vi "SPIN2_ODFT_iHV_w_Programmable_Delay.vi"(7 "Delay Time (s)":dbl=0.001 format="%#_13p", 9 "script name":string="ODFTwHV0", 10 "Ext_HV":dbl=38.0 format="%#_13g", 11 "Semiconductor Module Context":T1) -> (0 "error out":errorcluster)   [LabVIEW 2013]
uses:
  <vilib>/NI_TestStand_SemiconductorModule/NI_TestStand_Semiconductor_Module.lvlibp/PinMap/General/SemiconductorModuleContext.ctl
  <instrlib>/niHSDIO/niHSDIO.llb/niHSDIO_ctl Trigger Script - trigID Values (Ring).ctl
  <vilib>/NI_TestStand_SemiconductorModule/NI_TestStand_Semiconductor_Module.lvlibp/PinMap/DC Power/PinsToNIDCPowerSessions.vi
  <vilib>/NI_TestStand_SemiconductorModule/NI_TestStand_Semiconductor_Module.lvlibp/PinMap/Deprecated/PublishDataDoubleMultiplePinsMultipleInstruments.vi
  <vilib>/NI_TestStand_SemiconductorModule/NI_TestStand_Semiconductor_Module.lvlibp
panel:
  out "current measurements":dbl[][](array[numeric])
  out "Delta_iHV_Measurements":dbl[][](array[numeric])
  in  "Pins":string[](array[string])=["HV"]
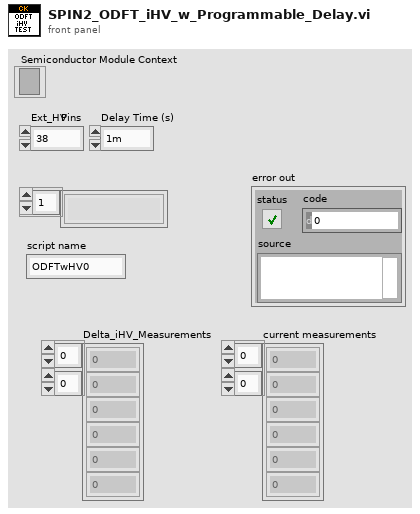
[diagram p1: front panel]
types:
  T1 = typedef "NI_TestStand_Semiconductor_Module.lvlibp/SemiconductorModuleContext.ctl" = refnum<k7>
  T2 = typedef "niHSDIO_ctl Trigger Script - trigID Values (Ring).ctl" = string
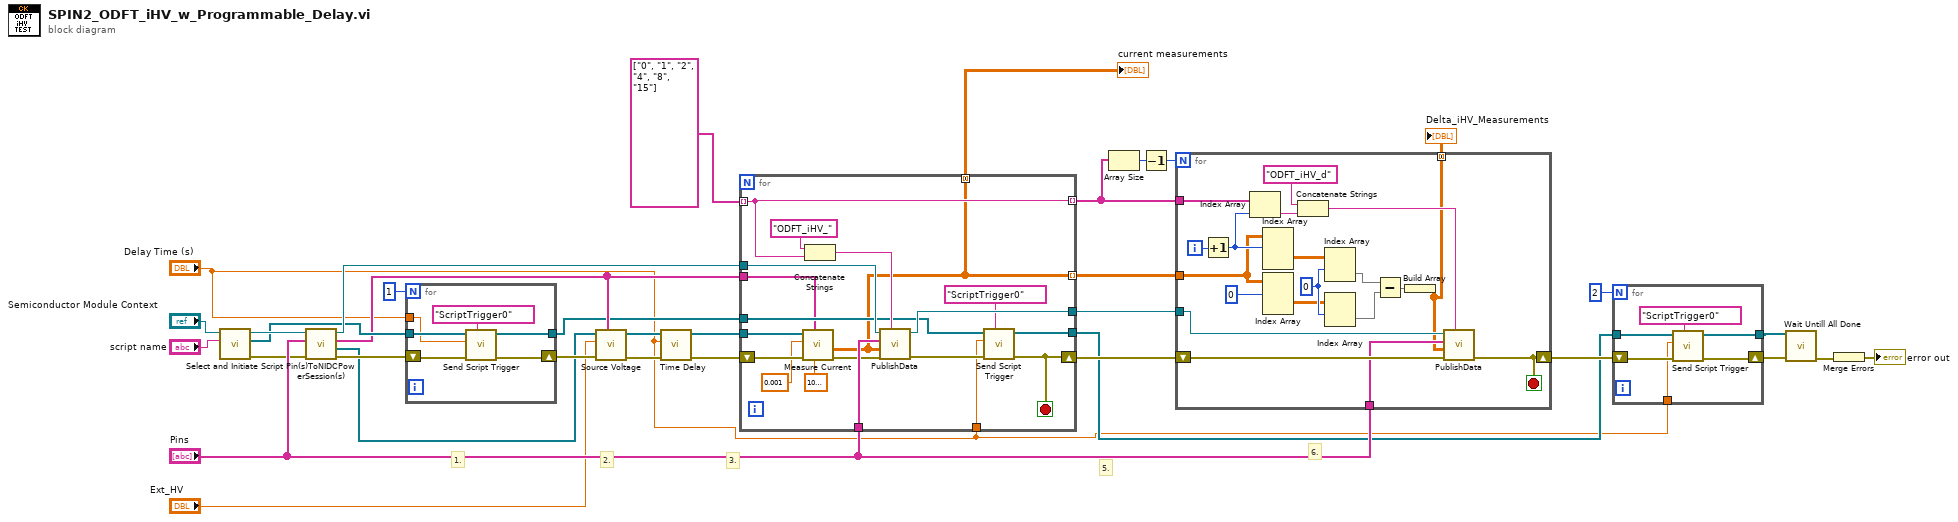
[diagram p0: block diagram]
diagram:
  # "3."
  # "6."
  # "5."
  # "2."
  # "1."
  n1 = call "Select and Initiate Script.vi"("script name"="script name", "Semiconductor Module Context"="Semiconductor Module Context") -> ("error out"=w17:errorcluster, "HSDIO GEN Sessions Out"=w18:refnum<k15>[], "Semiconductor Module Context Out"=w19:T1)  [unwired: 7 in]
  n2 = call-poly <vilib>:"Pin(s)ToNIDCPowerSession(s).vi"("error in (no error)"=w17, "Pins"="Pins", "Semiconductor Module Context"=w19) -> ("error out"=w33:errorcluster, "Instrument Sessions"=w16:refnum<k15>[], "Channel Lists"=w15:string[], "Semiconductor Module Context Out"=w21:T1)  [unwired: 4 in, 1 out]
  n3 = for {
    N: 1 -> [_]
    shift-right: [w38] -> w31
    shift-left: w33 -> [w39]
    tunnel: w18 -> [w37]
    tunnel: [w36] -> w13
    tunnel: "Delay Time (s)" -> [w35]
    n4 = call "Send Script Trigger.vi"("trigger id (script trigger 0)"=T2 "ScriptTrigger0", "error in (no error)"=w39, "Delay Time (s)"=w35, "HSDIO Sessions In"=w37) -> ("error out"=w38:errorcluster, "HSDIO Sessions Out"=w36:refnum<k15>[])  [unwired: 6 in]
  }
  n5 = call "Source Voltage.vi"("Channel Lists"=w15, "error in (no error)"=w31, "voltage level"="Ext_HV", "Instrument Sessions In"=w16) -> ("error out"=w11:errorcluster, "Instrument Sessions Out"=w30:refnum<k15>[])  [unwired: 4 in, 2 out]
  n6 = call "Time Delay"("error in (no error)"=w11, "Delay Time (s)"="Delay Time (s)") -> ("error out"=w10:errorcluster)  [unwired: 9 in]
  n7 = for {
    tunnel: string[] ["0", "1", "2", "4", "8", "15"] -> [w56] mode=indexing
    tunnel: w30 -> [w47]
    tunnel: w21 -> [w57]
    shift-right: [w50] -> w28
    shift-left: w10 -> [w49]
    tunnel: [w56] -> w26 mode=indexing
    tunnel: "Pins" -> [w55]
    tunnel: w13 -> [w51]
    tunnel: [w54] -> w23
    tunnel: w15 -> [w46]
    tunnel: [w41] -> w12 mode=indexing
    tunnel: [w43] -> w7
    tunnel: "Delay Time (s)" -> [w42]
    tunnel: [w41] -> w1 mode=concatenating
    stop <- w50 stop-if-true
    n8 = call "Measure Current.vi"("Result Multiplier"=1000000.0, "Channel Lists"=w46, "error in (no error)"=w49, "Delay Time (s)"=0.001, "DCPower Sessions In"=w47) -> ("error out"=w48:errorcluster, "current measurements"=w41:dbl[][])  [unwired: 4 in, 1 out]
    n9 = Concatenate Strings("ODFT_iHV_", w56) -> (w59:string)
    n10 = call-poly <vilib>:"PublishData.vi"("Measurement Id"=w59, "error in (no error)"=w48, "Data In"=w41, "Pins"=w55, "Semiconductor Module Context"=w57) -> ("error out"=w53:errorcluster, "Semiconductor Module Context Out"=w54:T1)  [unwired: 5 in]
    n11 = call "Send Script Trigger.vi"("trigger id (script trigger 0)"=T2 "ScriptTrigger0", "error in (no error)"=w53, "Delay Time (s)"=w42, "HSDIO Sessions In"=w51) -> ("error out"=w50:errorcluster, "HSDIO Sessions Out"=w43:refnum<k15>[])  [unwired: 6 in]
  }
  "current measurements" <- w1
  n12 = Array Size(array=w26) -> (size(s)=w25:i32)
  n13 = Decrement(x=w25) -> (x-1=w24:i32)
  n14 = for {
    N: w24 -> [_]
    tunnel: w26 -> [w75]
    shift-right: [w68] -> w8
    shift-left: w28 -> [w73]
    tunnel: "Pins" -> [w61]
    tunnel: w23 -> [w69]
    tunnel: w12 -> [w67]
    tunnel: [w60] -> w2 mode=concatenating
    i -> [w76]
    stop <- w68 stop-if-true
    w70 = 0 ("index (page)")
    n15 = Increment(x=w76) -> (x+1=w71:i32)
    n16 = Index Array(array=w75, index=w71) -> (element=w74:string)
    n17 = Index Array(array=w67, index (dim 0)=w71) -> (element=w66:dbl[][])  [unwired: 2 in]
    n18 = Index Array(array=w67, index (dim 0)=0 ("index (page)")) -> (element=w65:dbl[][])  [unwired: 2 in]
    n19 = Concatenate Strings("ODFT_iHV_d", w74) -> (w77:string)
    n20 = Index Array(array=w66, index (row)=w70) -> (element=w63:dbl[])  [unwired: 1 in]
    n21 = Index Array(array=w65, index (row)=w70) -> (element=w64:dbl[])  [unwired: 1 in]
    n22 = Subtract(x=w63, y=w64) -> (x-y=w62:dbl[])
    n23 = Build Array(w62) -> (w60:dbl[][])
    n24 = call-poly <vilib>:"PublishData.vi"("Measurement Id"=w77, "error in (no error)"=w73, "Data In"=w60, "Pins"=w61, "Semiconductor Module Context"=w69) -> ("error out"=w68:errorcluster)  [unwired: 5 in, 1 out]
  }
  "Delta_iHV_Measurements" <- w2
  n25 = for {
    N: 2 -> [_]
    shift-right: [w82] -> w5
    shift-left: w8 -> [w83]
    tunnel: w7 -> [w81]
    tunnel: [w80] -> w6
    tunnel: "Delay Time (s)" -> [w79]
    n26 = call "Send Script Trigger.vi"("trigger id (script trigger 0)"=T2 "ScriptTrigger0", "error in (no error)"=w83, "Delay Time (s)"=w79, "HSDIO Sessions In"=w81) -> ("error out"=w82:errorcluster, "HSDIO Sessions Out"=w80:refnum<k15>[])  [unwired: 6 in]
  }
  n27 = call "Wait Untill All Done.vi"("error in (no error)"=w5, "HSDIO Sessions In"=w6) -> ("error out"=w14:errorcluster)  [unwired: 8 in, 1 out]
  n28 = Merge Errors(w14) -> (→"error out":errorcluster)
